vi "Roughness.vi"(7 "Data":dbl[](array[numeric]), 11 "Sub Sampling Interval (10)":i32=10) -> (1 "Mean":dbl, 3 "RMS":dbl, 4 "Skewdness":dbl, 6 "Kurtosis":dbl, 10 "RzDIN":dbl, 12 "Max":dbl, 13 "Min":dbl, 14 "Max P-P":dbl, 15 "RzJIS":dbl)   [LabVIEW 2018]
uses:
  08642fd6-f559-4f98-a88d-f53b29b0be6c.vi
  7bec75e6-5c25-4f8a-84bb-4e4617cdde0c.vi
  <vilib>/Analysis/5stat.llb/RMS (DBL).vi
  <vilib>/Analysis/baseanly.llb/Mean (DBL).vi
  3c222fba-c6c0-45ca-b7e9-bc0cb2a739ce.vi
  08642fd6-f559-4f98-a88d-f53b29b0be6c.vi/4577ad6d-6a06-4f88-9475-352725b0b4ed.vi
  08642fd6-f559-4f98-a88d-f53b29b0be6c.vi/5b938a84-013f-4cec-9e5d-96a1874184e0.vi
  3c222fba-c6c0-45ca-b7e9-bc0cb2a739ce.vi/40775d3b-a039-4f9e-95aa-fd5165530a9a.vi
  3c222fba-c6c0-45ca-b7e9-bc0cb2a739ce.vi/2d12377d-1c31-425e-821c-bece12dc1f52.vi
  <vilib>/Analysis/NI_AALBase.lvlib
  <vilib>/Analysis/NI_AALPro.lvlib
  <vilib>/gmath/NI_Gmath.lvlib
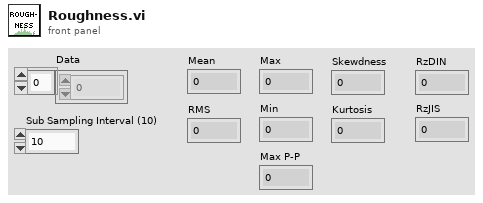
[diagram p1: front panel]
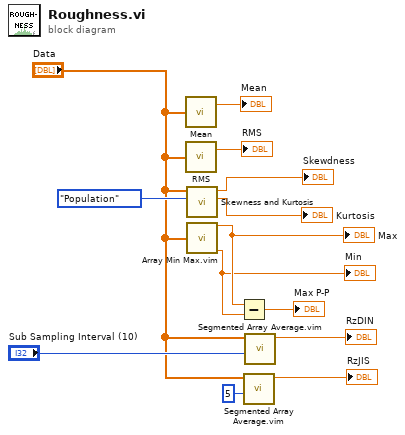
[diagram p0: block diagram]
diagram:
  n1 = call-poly <vilib>:"Mean.vi"("X"="Data") -> ("mean"=→"Mean":dbl)  [unwired: 1 out]
  n2 = call-poly <vilib>:"RMS.vi"("X"="Data") -> ("rms value"=→"RMS":dbl)  [unwired: 1 out]
  n3 = call <vilib>:"Skewness and Kurtosis.vi"("Weighting (Sample)"=enum16{"Sample", "Population"}."Population", "X"="Data") -> ("kurtosis"=→"Kurtosis":dbl, "skewness"=→"Skewdness":dbl)  [unwired: 7 in, 1 out]
  n4 = call "Array Min Max.vim"("Array"="Data") -> ("Max"=w8:dbl, "Min"=w7:dbl)  [unwired: 13 in]
  "Max" <- w8
  "Min" <- w7
  n5 = Subtract(x=w8, y=w7) -> (x-y=→"Max P-P":dbl)
  n6 = call "Segmented Array Average.vim"("Sub Sampling Interval"=5, "Data"="Data") -> ("Segmented Average"=→"RzJIS":dbl)  [unwired: 9 in]
  n7 = call "Segmented Array Average.vim"("Sub Sampling Interval"="Sub Sampling Interval (10)", "Data"="Data") -> ("Segmented Average"=→"RzDIN":dbl)  [unwired: 9 in]
